vi "OC2 Setup Output.vi"(3 "error in (no error)":errorcluster, 4 "output report in":T1 {"Output freq." format="%.1f"; "Output" items=["Negative", "Positive"]}, 5 "enable":bool, 6 "VISA resource name":refnum<visa-resource-name>) -> (0 "error out":errorcluster, 1 "output report out":T1 {"Output freq." format="%.1f"; "Output" items=["Negative", "Positive"]}, 2 "dup VISA resource name":refnum<visa-resource-name>)   [LabVIEW 2009]
doc: "TCM Setup Output.vi\n\nVI that sets the output information, accepts a cluster that contains the following variables:\nOutput - negative or positive output\nOutput min % - minimum output percentage allowed\nOutput max % - maximum output percentage allowed\nOutput freq - frequency of the PWM output signal\n\nCOPYRIGHT ELECTRON DYNAMICS LTD"
panel:
  out "write data":string
  # "Setup output variables"
  # "V1.02"
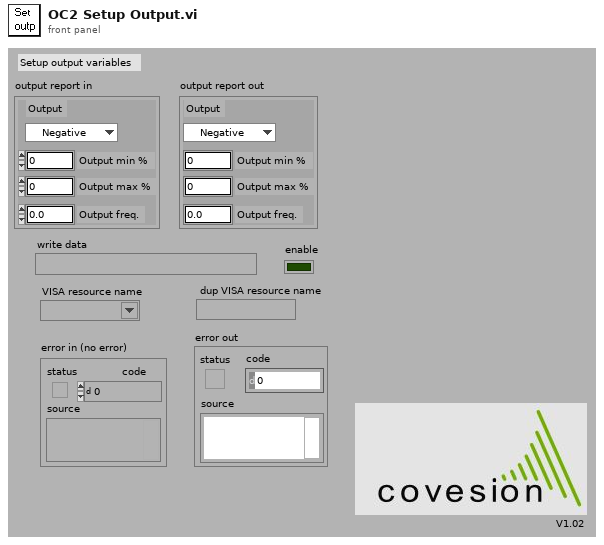
[diagram p1: front panel]
types:
  T1 = cluster{"Output":u16, "Output min %":dbl, "Output max %":dbl, "Output freq.":dbl}
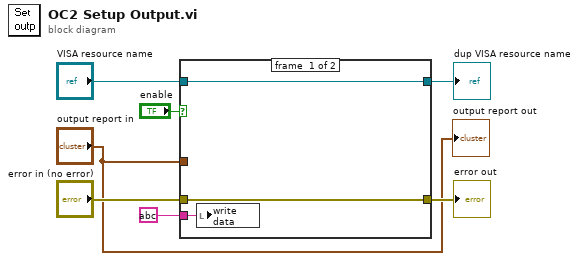
[diagram p0: block diagram]
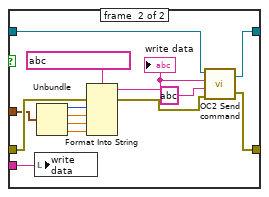
[diagram p2: hidden frame]
diagram:
  n1 = case shown="True" "enable" {
    tunnel: "VISA resource name" -> [w10 w21]
    tunnel: "error in (no error)" -> [w9 w20]
    tunnel: [w9 w17] -> w4
    tunnel: [w10 w19] -> w3
    tunnel: "output report in" -> [_ w16]
    tunnel: string ? -> [w8 w11]
    frame #0 {
      n2 = local write "write data"(w8) -> ()
    }
    frame #1 {
      n3 = local write "write data"(w11) -> ()
      n4 = Unbundle(w16) -> ("Output"=w15:u16, "Output min %"=w14:dbl, "Output max %"=w13:dbl, "Output freq."=w12:dbl)
      n5 = Format Into String(format string=string ?, error in=w20, w15, w14, w13, w12) -> (resulting string=w22:string, error out=w18:errorcluster)  [unwired: 1 in]
      "write data" <- w22
      n6 = call "OC2 Send command.vi"("VISA resource name"=w21, "Command data"=w22, "Command"=string ?, "error in (no error)"=w18) -> ("dup VISA resource name"=w19:refnum<visa-resource-name>, "error out"=w17:errorcluster)  [unwired: 1 in]
    }
  }
  "dup VISA resource name" <- w3
  "error out" <- w4
  "output report out" <- "output report in"
